vi "Text-Get Size.vi"(0 "String":refnum<vi>, 7 "Text":string, 11 "error in (no error)":errorcluster) -> (4 "reference out":refnum<vi>, 6 "width":i16, 8 "height":i16, 15 "error out":errorcluster)   [LabVIEW 2015]
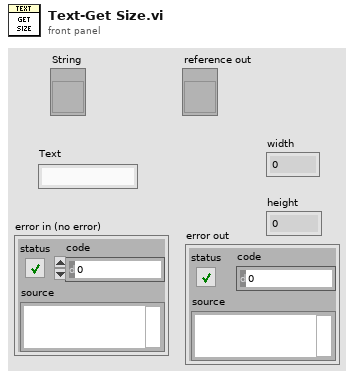
[diagram p1: front panel]
types:
  T1 = enum16{"User-specified Font", "Application Font", "System Font", "Dialog Font"}
  T2 = cluster{"Font Name:":string, "Size":i16, "Strikeout?":bool, "Italic?":bool, "Underline?":bool, "Outline?":bool, "Shadow?":bool, "Bold?":bool}
  T3 = typedef "LVFontTypeDef.ctl" = cluster{"Font Name":string, "Size":u16, "Bold":bool, "Italic":bool, "Underline":bool, "Strikeout":bool, "Color":u32}
  T4 = cluster{"left":i16, "top":i16, "right":i16, "bottom":i16}
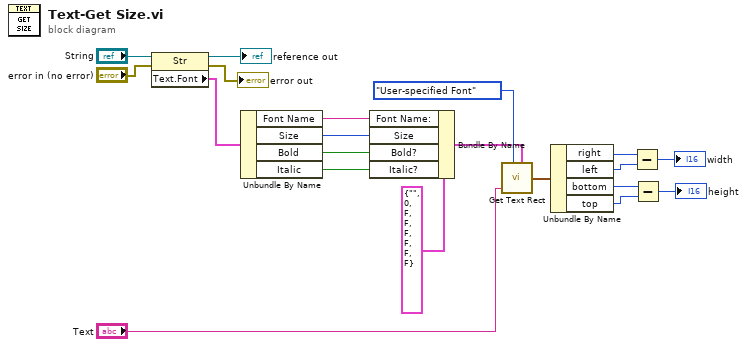
[diagram p0: block diagram]
diagram:
  n1 = property class="Str"(reference="String", error in="error in (no error)") -> (reference out=→"reference out":refnum<vi>, error out=→"error out":errorcluster, "Text.Font"=w18:T3)
  n2 = Unbundle By Name(w18) -> ("Font Name"=w17:string, "Size"=w15:u16, "Bold"=w14:bool, "Italic"=w13:bool)
  n3 = Bundle By Name(cluster=T2 {"Font Name:"="", "Size"=0, "Strikeout?"=FALSE, "Italic?"=FALSE, "Underline?"=FALSE, "Outline?"=FALSE, "Shadow?"=FALSE, "Bold?"=FALSE} ("[user-specified font]"), "Font Name:"=w17, "Size"=w15, "Bold?"=w14, "Italic?"=w13) -> (w1:T2)
  n4 = call <vilib>:"Get Text Rect.vi"("desired font(Application)"=T1."User-specified Font", "text"="Text", "[user-specified font]"=w1) -> ("rect"=w11:T4)  [unwired: 6 in]
  n5 = Unbundle By Name(w11) -> ("right"=w10:i16, "left"=w9:i16, "bottom"=w8:i16, "top"=w7:i16)
  n6 = Subtract(x=w10, y=w9) -> (x-y=→"width":i16)
  n7 = Subtract(x=w8, y=w7) -> (x-y=→"height":i16)
